vi "GA Crd Data.vi"(8 "error in (no error)":errorcluster caption="错误输入（无错误）", 9 "FifoIndex":i16, 10 "pCrdData":u32, 11 "nCrdNum":i16) -> (0 "error out":errorcluster caption="错误输出", 2 "pCrdData out":u32, 3 "function return":i32)   [LabVIEW 2015, in "GAS.lvlib"]
doc: "extern \"C\" __declspec(dllimport) int GA_CrdData(short nCrdNum,void *pCrdData,short FifoIndex=0);"
uses:
  <userlib>/BP_GAS/GAS.lvlib
  <userlib>/BP_GAS/GAS.dll
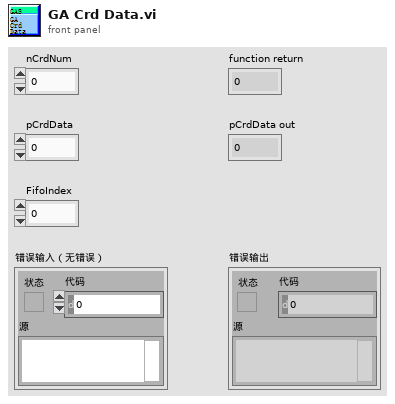
[diagram p1: front panel]
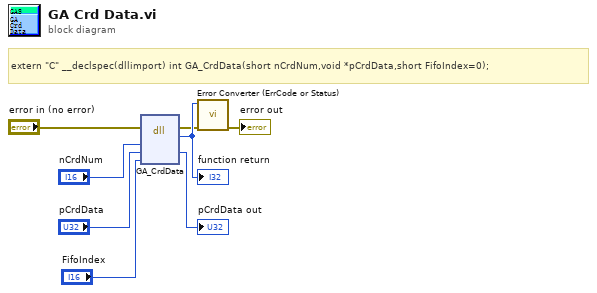
[diagram p0: block diagram]
diagram:
  # "extern \"C\" __declspec(dllimport) int GA_CrdData(short nCrdNum,void *pCrdData,short FifoIndex=0);"
  n1 = dll-call lib="E:/Program Files (x86)/National Instruments/LabVIEW 2015/user.lib/BP_GAS/GAS.*" fn="GA_CrdData"(error in="error in (no error)", "nCrdNum"="nCrdNum", "pCrdData"="pCrdData", "FifoIndex"="FifoIndex") -> (error out=w2:errorcluster, w8:i32, "pCrdData"=→"pCrdData out":u32)  [unwired: 4 in, 1 out]
  "function return" <- w8
  n2 = call "Error Converter (ErrCode or Status).vi"("error in (no error)"=w2, "error code"=w8) -> ("error out"=→"error out":errorcluster)  [unwired: 9 in]
